vi "modbus input.vi"(8 "error in (no error)":errorcluster, 10 "data table in":T1, 11 "Modbus Module runtime in":refnum<class "Modbus Module runtime.lvclass">) -> (0 "error out":errorcluster, 2 "data table out":T1, 3 "Modbus Module runtime out":refnum<class "Modbus Module runtime.lvclass">)   [LabVIEW 2015, in "Modbus Module runtime.lvclass"]
uses:
  Modbus Module runtime.lvclass
  <vilib>/NI/Tag Bus/table/data table.ctl
  Modbus Module runtime.lvclass/Modbus Module runtime.ctl
  <vilib>/NI/Modbus Library/API/Modbus API.lvclass
  <vilib>/NI/Tag Bus/table/data table.lvlib
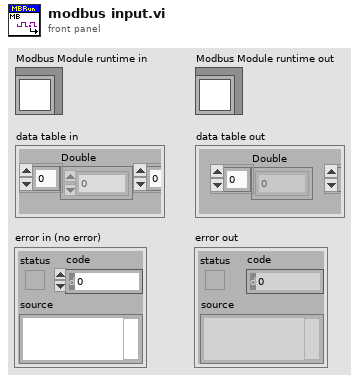
[diagram p1: front panel]
types:
  T1 = typedef "tag bus.lvlib/data table.lvlib/data table.ctl" = cluster{"Double":dbl[], "Single":sgl[], "I64":i64[], "I32":i32[], "I16":i16[], "I8":i8[], "U64":u64[], "U32":u32[], "U16":u16[], "U8":u8[], "Boolean":bool[], "String":string[], "Array of Double":cluster{"DBL Array":dbl[]}[], "Array of Single":cluster{"SGL Array":sgl[]}[], "Array of I64":cluster{"I64 Array":i64[]}[], "Array of I32":cluster{"I32 Array":i32[]}[], "Array of I16":cluster{"I16 Array":i16[]}[], "Array of I8":cluster{"I8 Array":i8[]}[], "Array of U64":cluster{"U64 Array":u64[]}[], "Array of U32":cluster{"U32 Array":u32[]}[], "Array of U16":cluster{"U16 Array":u16[]}[], "Array of U8":cluster{"U8 Array":u8[]}[], "Array of Boolean":cluster{"Boolean Array":bool[]}[], "Array of String":cluster{"String Array":string[]}[]}
  T2 = typedef "Modbus Module runtime.lvclass/bulk data access.ctl" = cluster{"modbus type":T3, "start":u16, "length":u16, "maps":T4[]}
  T3 = typedef "Modbus Module Channel.lvclass/data bank type.ctl" = enum16{"Coils", "Discrete Inputs", "Input Registers", "Holding Registers"}
  T4 = typedef "Modbus Module runtime.lvclass/data mapping elements.ctl" = cluster{"data type":T5, "data index":i32, "element index":i32, "subindex/regcount":i32}
  T5 = typedef "tag bus.lvlib/tag descriptor.lvclass/Data Type.ctl" = enum16{"Double", "Single", "I64", "I32", "I16", "I8", "U64", "U32", "U16", "U8", "Boolean", "String", "Array of Double", "Array of Single", "Array of I64", "Array of I32", "Array of I16", "Array of I8", "Array of U64", "Array of U32", "Array of U16", "Array of U8", "Array of Boolean", "Array of String"}
  T6 = cluster{"32-bit: first word low":bool, "64-bit: first dword low":bool}
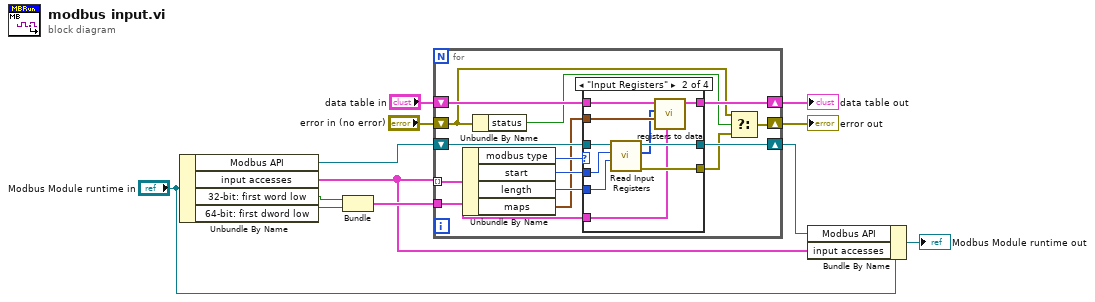
[diagram p0: block diagram]
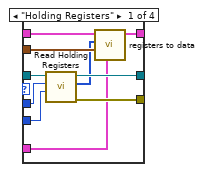
[diagram p2: hidden frame]
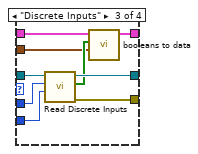
[diagram p3: hidden frame]
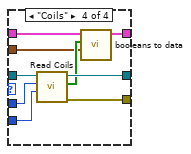
[diagram p4: hidden frame]
diagram:
  n1 = Unbundle By Name("Modbus Module runtime in") -> ("Modbus API"=w3:refnum<class "Modbus API.lvclass">, "input accesses"=w9:T2[], "32-bit: first word low"=w10:bool, "64-bit: first dword low"=w11:bool)
  n2 = Bundle("32-bit: first word low"=w10, "64-bit: first dword low"=w11) -> (w12:T6)  [unwired: 1 in]
  n3 = for {
    shift-right: [w24] -> w4
    shift-left: w3 -> [w25]
    shift-right: [w26] -> w6
    shift-left: "error in (no error)" -> [w15]
    tunnel: w9 -> [w22] mode=indexing
    shift-right: [w17] -> w8
    shift-left: "data table in" -> [w18]
    tunnel: w12 -> [w13]
    n4 = Unbundle By Name(w22) -> ("modbus type"=w19:T3, "start"=w20:u16, "length"=w21:u16, "maps"=w16:T4[])
    n5 = Unbundle By Name(w15) -> ("status"=w14:bool)
    n6 = case shown="\"Input Registers\"" w19 {
      tunnel: w25 -> [w34 w44 w53 w62]
      tunnel: [w36 w46 w55 w64] -> w24
      tunnel: [w35 w45 w54 w63] -> w23
      tunnel: w20 -> [w33 w43 w52 w61]
      tunnel: w21 -> [w32 w42 w51 w60]
      tunnel: w18 -> [w31 w41 w50 w58]
      tunnel: [w30 w40 w49 w59] -> w17
      tunnel: w16 -> [w29 w39 w47 w56]
      tunnel: w13 -> [w27 w37 _ _]
      frame "Holding Registers" {
        n7 = call-dynamic "Read Holding Registers.vi"("number of inputs"=w32, "starting address"=w33, "Modbus instance in"=w34) -> ("error out"=w35:errorcluster, "register values"=w28:u16[], "Modbus instance out"=w36:refnum<class "Modbus API.lvclass">)  [unwired: 6 in]
        n8 = call "registers to data.vi"("word order"=w27, "specifications"=w29, "registers"=w28, "allocation"=w31) -> ("data table"=w30:T1)  [unwired: 7 in]
      }
      frame "Input Registers" {
        n9 = call-dynamic "Read Input Registers.vi"("number of inputs"=w42, "starting address"=w43, "Modbus instance in"=w44) -> ("error out"=w45:errorcluster, "register values"=w38:u16[], "Modbus instance out"=w46:refnum<class "Modbus API.lvclass">)  [unwired: 6 in]
        n10 = call "registers to data.vi"("word order"=w37, "specifications"=w39, "registers"=w38, "allocation"=w41) -> ("data table"=w40:T1)  [unwired: 7 in]
      }
      frame "Discrete Inputs" {
        n11 = call-dynamic "Read Discrete Inputs.vi"("number of inputs"=w51, "starting address"=w52, "Modbus instance in"=w53) -> ("error out"=w54:errorcluster, "discrete inputs"=w48:bool[], "Modbus instance out"=w55:refnum<class "Modbus API.lvclass">)  [unwired: 6 in]
        n12 = call "booleans to data.vi"("specifications"=w47, "booleans"=w48, "allocation"=w50) -> ("data table"=w49:T1)  [unwired: 8 in]
      }
      frame "Coils" {
        n13 = call-dynamic "Read Coils.vi"("number of inputs"=w60, "starting address"=w61, "Modbus instance in"=w62) -> ("error out"=w63:errorcluster, "coils"=w57:bool[], "Modbus instance out"=w64:refnum<class "Modbus API.lvclass">)  [unwired: 6 in]
        n14 = call "booleans to data.vi"("specifications"=w56, "booleans"=w57, "allocation"=w58) -> ("data table"=w59:T1)  [unwired: 8 in]
      }
    }
    n15 = Select(t=w15, s=w14, f=w23) -> (s? t:f=w26:errorcluster)
  }
  "error out" <- w6
  "data table out" <- w8
  n16 = Bundle By Name(cluster="Modbus Module runtime in", "Modbus API"=w4, "input accesses"=w9) -> (→"Modbus Module runtime out":refnum<class "Modbus Module runtime.lvclass">)
